vi "ws DB Open.vi"(8 "error in (no error)":errorcluster, 11 "DB Path (empty - use default)":path) -> (0 "error out":errorcluster, 3 "Connection Refnum":T1)   [LabVIEW 2011]
uses:
  SI.LIB/ODBC/SQL Controls/Connection Refnum.ctl
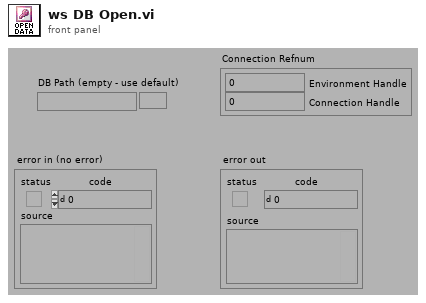
[diagram p1: front panel]
types:
  T1 = typedef "Connection Refnum.ctl" = cluster{"Environment Handle":i32, "Connection Handle":i32}
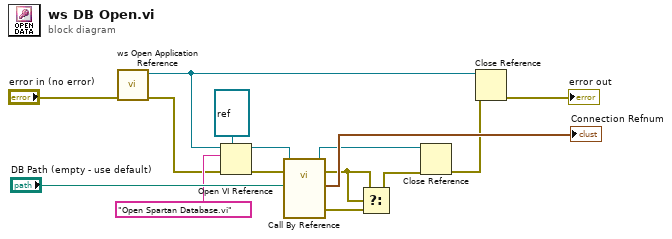
[diagram p0: block diagram]
diagram:
  n1 = call "ws Open Application Reference.vi"("error in (no error)"="error in (no error)") -> ("error out"=w2:errorcluster, "application reference"=w1:refnum<vi>)  [unwired: 9 in]
  n2 = Open VI Reference(type specifier VI Refnum (for type only)=refnum<vi> refnum, application reference (local)=w1, vi path="Open Spartan Database.vi", error in (no error)=w2) -> (vi reference=w11:refnum<vi>, error out=w12:errorcluster)  [unwired: 2 in]
  n3 = call-by-ref "?"(reference=w11, error in=w12, "DB Path (empty - use default)"="DB Path (empty - use default)") -> (reference out=w7:refnum<vi>, error out=w8:errorcluster, 0:"error out"=w9:errorcluster, "Connection Refnum"=→"Connection Refnum":T1)  [unwired: 9 in]
  n4 = Select(t=w8, s=w8, f=w9) -> (s? t:f=w6:errorcluster)
  n5 = Close Reference(reference=w7, error in (no error)=w6) -> (error out=w5:errorcluster)
  n6 = Close Reference(reference=w1, error in (no error)=w5) -> (error out=→"error out":errorcluster)
